vi "Analyze.vi"(8 "error in (no error)":errorcluster, 10 "Image in":T1, 11 "Analyze Distanz in":refnum<class "Analyze Distanz.lvclass">) -> (0 "error out":errorcluster, 1 "Result":refnum<class "Analyze Results Base.lvclass">, 2 "Image out":T1, 3 "Analyze Distanz out":refnum<class "Analyze Distanz.lvclass">)   [LabVIEW 2014, in "Analyze.lvlib" / "Analyze Distanz.lvclass"]
uses:
  Analyze Distanz.lvclass
  <vilib>/vision/Image Controls.llb/IMAQ Image.ctl
  Results and Overlays/Results Base/Analyze Results Base.lvclass
  Results and Overlays/Results Distance/Analyze Results Distanz.lvclass
  Results and Overlays/Results Distance/Analyze Results Distanz.lvclass/Analyze Results Distanz.ctl
  Results and Overlays/Results Distance/Write Distances.vi
  Results and Overlays/Results Distance/Write Overlay Positions.vi
  Analyze BaseClass/Analyze BaseClass/Analyze BaseClass.lvclass
  Utility/POLARIS Vision utility.lvlib
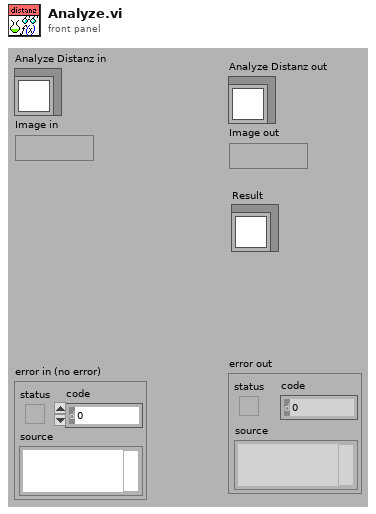
[diagram p1: front panel]
types:
  T1 = typedef "IMAQ Image.ctl" = refnum<image>
  T2 = typedef "ROI Descriptor" = cluster{"Global Rectangle":i32[], "Contours":cluster{"ID":enum32{"External", "Internal"}, "Type":u32, "Coordinates":i32[]}[]}
  T3 = cluster{"ID":enum32{"External", "Internal"}, "Type":u32, "Coordinates":i32[]}[]
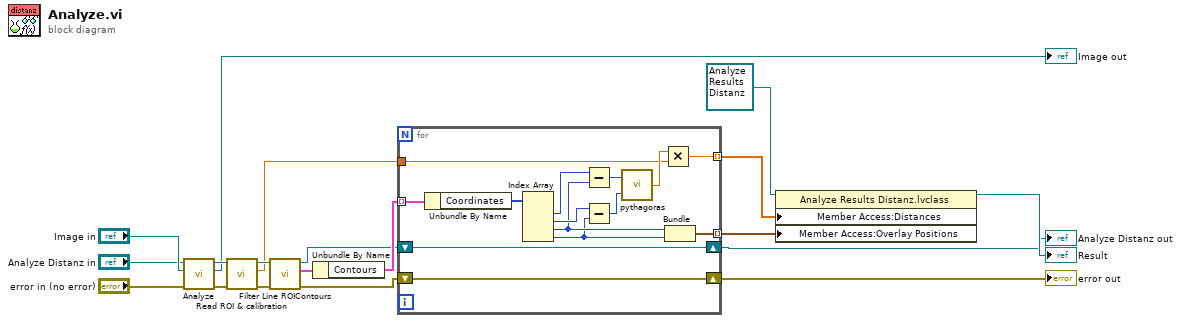
[diagram p0: block diagram]
diagram:
  n1 = call-parent "Analyze.vi"("error in (no error)"="error in (no error)", "Image in"="Image in", "Analyze BaseClass in"="Analyze Distanz in") -> ("error out"=w9:errorcluster, "Image out"=→"Image out":T1, "Analyze BaseClass out"=w10:refnum<class "Analyze Distanz.lvclass">)  [unwired: 5 in, 1 out]
  n2 = call-dynamic "Read ROI & calibration.vi"("error in (no error)"=w9, "Analyze BaseClass in"=w10) -> ("error out"=w19:errorcluster, "calibration mm/px"=w15:dbl[unit], "Analyze BaseClass out"=w18:refnum<class "Analyze Distanz.lvclass">)  [unwired: 6 in, 1 out]
  n3 = call-dynamic "Filter Line ROIContours.vi"("error in (no error)"=w19, "Analyze BaseClass in"=w18) -> ("error out"=w13:errorcluster, "Line contours"=w17:T2, "Analyze BaseClass out"=w14:refnum<class "Analyze Distanz.lvclass">)  [unwired: 7 in]
  n4 = Unbundle By Name(w17) -> ("Contours"=w16:T3)
  n5 = for {
    tunnel: w16 -> [w33] mode=indexing
    tunnel: w15 -> [w26]
    shift-right: [w25] -> w3
    shift-left: w14 -> [w25]
    shift-right: [w24] -> w12
    shift-left: w13 -> [w24]
    tunnel: [w20] -> w6 mode=indexing
    tunnel: [w21] -> w5 mode=indexing
    n6 = Unbundle By Name(w33) -> ("Coordinates"=w32:i32[])
    n7 = Index Array(array=w32) -> (element #1=w30:i32, element #2=w29:i32, element #3=w23:i32, element #4=w22:i32)  [unwired: 4 in]
    n8 = Subtract(x=w30, y=w23) -> (x-y=w31:i32)
    n9 = Subtract(x=w29, y=w22) -> (x-y=w28:i32)
    n10 = call "pythagoras.vi"("b"=w28, "a"=w31) -> ("c"=w27:dbl)
    n11 = Multiply(x=w27, y=w26) -> (x*y=w20:dbl[unit])
    n12 = Bundle(w23, w22) -> (w21:cluster{i32, i32})  [unwired: 1 in]
  }
  "error out" <- w12
  "Analyze Distanz out" <- w3
  n13 = property class="Analyze Results Distanz.lvclass"(reference=refnum<class "Analyze Results Distanz.lvclass"> refnum ("Analyze Results Distanz.lvclass"), "Member Access:Distances"=w6, "Member Access:Overlay Positions"=w5) -> (reference out=→"Result":refnum<class "Analyze Results Distanz.lvclass">)  [unwired: 1 in, 1 out]
